vi "Generate Sine.vi"(10 "brightness":dbl, 11 "period (ms)":u32) -> (3 "sine":i32[](array[numeric]))   [LabVIEW 2025]
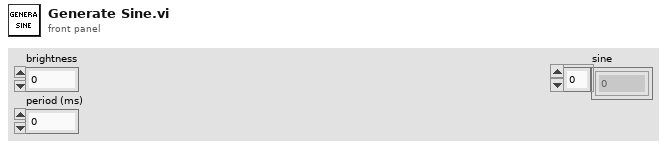
[diagram p1: front panel]
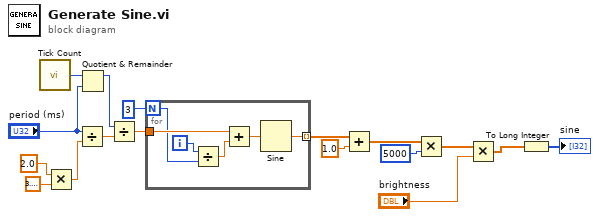
[diagram p0: block diagram]
diagram:
  n1 = call "Tick Count"() -> ("Tick Count(mSec)"=w14:u32)
  n2 = Multiply(x=2.0, y=3.141592653589793) -> (x*y=w4:dbl)
  n3 = Divide(x="period (ms)", y=w4) -> (x/y=w1:dbl)
  n4 = Quotient & Remainder(x=w14, y="period (ms)") -> (x-y*floor(x/y)=w12:u32)  [unwired: 1 out]
  n5 = Divide(x=w12, y=w1) -> (x/y=w13:dbl)
  n6 = for {
    N: 3 -> [w21]
    tunnel: w13 -> [w23]
    tunnel: [w18] -> w11 mode=indexing
    i -> [w22]
    n7 = Divide(x=w22, y=w21) -> (x/y=w19:dbl)
    n8 = Add(x=w23, y=w19) -> (x+y=w20:dbl)
    n9 = Sine(x=w20) -> (sin(x)=w18:dbl)
  }
  n10 = Add(x=w11, y=1.0) -> (x+y=w7:dbl[])
  n11 = Multiply(x=w7, y=5000) -> (x*y=w9:dbl[])
  n12 = Multiply(x=w9, y="brightness") -> (x*y=w16:dbl[])
  n13 = To Long Integer(number=w16) -> (32bit integer=→"sine":i32[])
